vi "FakeSignalGenerator(OptimzerDebug).vi"(8 "Z":dbl, 9 "Y":dbl=1.0, 10 "X":dbl) -> (2 "E":dbl)   [LabVIEW 2014, in "GenericDAQ.lvlib"]
doc: "This template is the starting point for creating a model function to be passed to the Nonlinear Curve Fit.vi."
uses:
  <instrlib>/GenericDAQ/GenericDAQ.lvlib
  <instrlib>/GenericDAQ/VI/InstrParams.vi
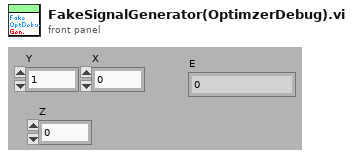
[diagram p1: front panel]
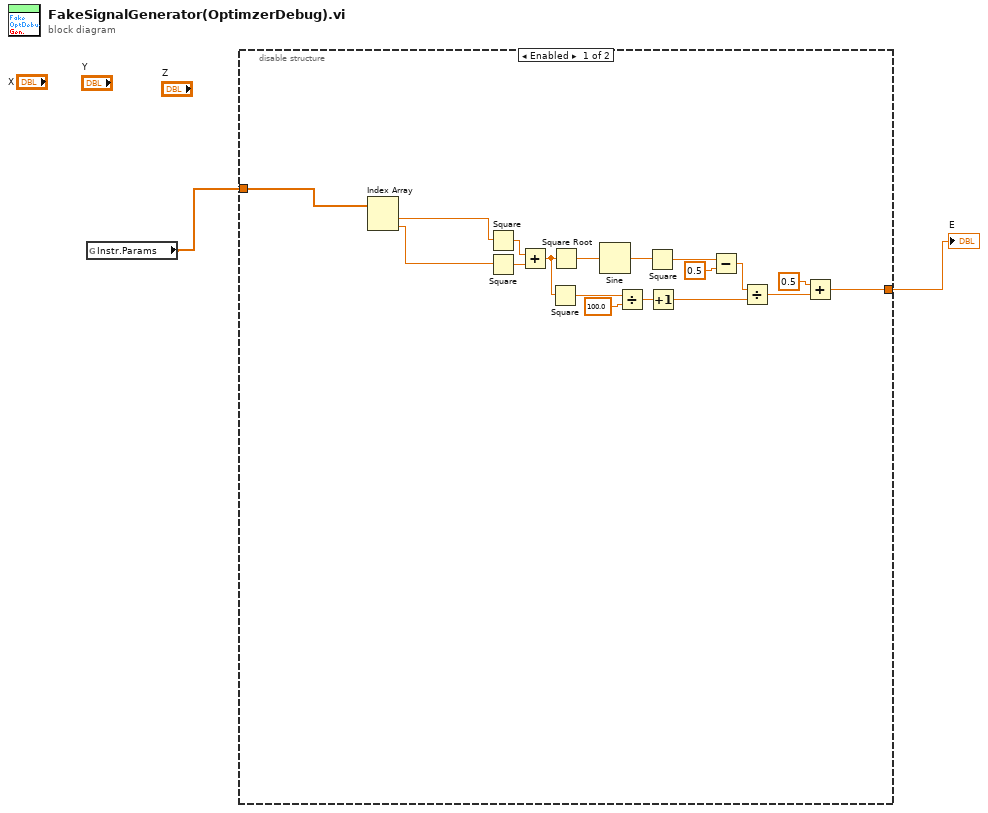
[diagram p0: block diagram]
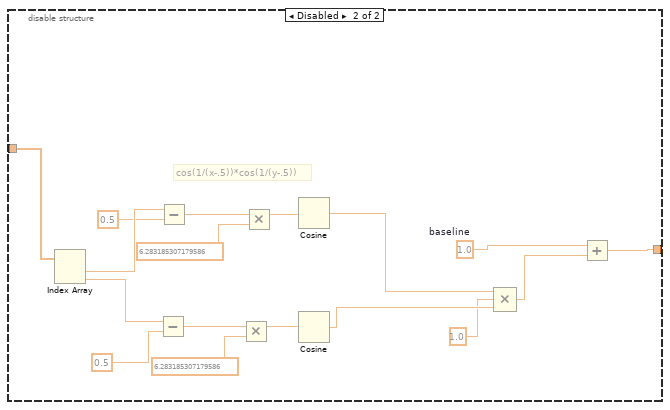
[diagram p2: hidden frame]
diagram:
  n1 = global read "InstrParams.vi" "Instr.Params"() -> (w2:dbl[])
  n2 = disable-structure shown="Enabled" {
    disable-tunnel: w2 -> [w3 w21]
    disable-tunnel: [w4 w22] -> w1
    frame Enabled {
      n3 = Index Array(array=w3) -> (element #1=w5:dbl, element #2=w6:dbl)  [unwired: 2 in]
      n4 = Square(x=w5) -> (x^2=w8:dbl)
      n5 = Square(x=w6) -> (x^2=w7:dbl)
      n6 = Add(x=w8, y=w7) -> (x+y=w9:dbl)
      n7 = Square(x=w9) -> (x^2=w15:dbl)
      n8 = Square Root(x=w9) -> (sqrt(x)=w10:dbl)
      n9 = Sine(x=w10) -> (sin(x)=w11:dbl)
      n10 = Divide(x=w15, y=100.0) -> (x/y=w17:dbl)
      n11 = Square(x=w11) -> (x^2=w12:dbl)
      n12 = Increment(x=w17) -> (x+1=w18:dbl)
      n13 = Subtract(x=w12, y=0.5) -> (x-y=w14:dbl)
      n14 = Divide(x=w14, y=w18) -> (x/y=w19:dbl)
      n15 = Add(x=0.5, y=w19) -> (x+y=w4:dbl)
    }
    frame Disabled {
      w24 = 1.0  # baseline
      # "cos(1/(x-.5))*cos(1/(y-.5))"
      n16 = Index Array(array=w21) -> (element #1=w36:dbl, element #2=w37:dbl)  [unwired: 2 in]
      n17 = Subtract(x=w37, y=0.5 ("focus_pos")) -> (x-y=w29:dbl)
      n18 = Subtract(x=w36, y=0.5 ("focal plane pos")) -> (x-y=w28:dbl)
      n19 = Multiply(x=w29, y=6.283185307179586) -> (x*y=w32:dbl)
      n20 = Multiply(x=w28, y=6.283185307179586) -> (x*y=w33:dbl)
      n21 = Cosine(x=w33) -> (cos(x)=w30:dbl)
      n22 = Cosine(x=w32) -> (cos(x)=w31:dbl)
      n23 = Compound Arithmetic op=MULTIPLY(w30, 1.0 ("value"), w31) -> (w23:dbl)
      n24 = Add(x=w24, y=w23) -> (x+y=w22:dbl)
    }
  }
  "E" <- w1
